vi "Fluke 5080 Resistance Calibrator.vi"() -> ()   [LabVIEW 2012]
doc: "This example shows how to configure the calibrator to resistance output mode."
uses:
  <instrlib>/Fluke 5080/Fluke 5080.lvlib
panel:
  in  "Resistance (1900.0 Ohm)":dbl=1900.0
  in  "Impedance Compensation (0: None)":i32(ring) items=["None", "2-wire", "4-wire"]
  in  "Serial Configuration":T1={"Baud Rate"=9600, "Parity"=0, "Data Bits"=8, "Stop Bits"=10, "Flow Control"=0} {"Flow Control" items=["None", "XON/XOFF", "RTS/CTS", "XON/XOFF & RTS/CTS", "DTR/DSR", "XON/XOFF & DTR/DSR"]; "Stop Bits" items=["1.0"=10, "1.5"=15, "2.0"=20]; "Data Bits" items=["7"=7, "8"=8]; "Parity" items=["None", "Odd", "Even", "Mark", "Space"]; "Baud Rate" items=["300"=300, "600"=600, "1200"=1200, "2400"=2400, "4800"=4800, "9600"=9600, "19200"=19200]}
  in  "VISA resource name":refnum<visa-resource-name>
  in  "Output Type (0: DC Volts)":i32(ring)=8 items=["DC Volts", "AC Volts", "DC Current", "AC Current", "DC Power", "AC Power", "Dual DC Volts", "Dual AC Volts", "Resistance"]
  # "(c) 2010 National Instruments.  ALL RIGHTS RESERVED."
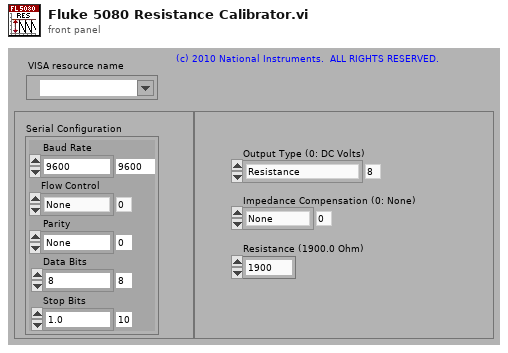
[diagram p1: front panel]
types:
  T1 = cluster{"Baud Rate":u32, "Parity":u16, "Data Bits":u16, "Stop Bits":u16, "Flow Control":u16}
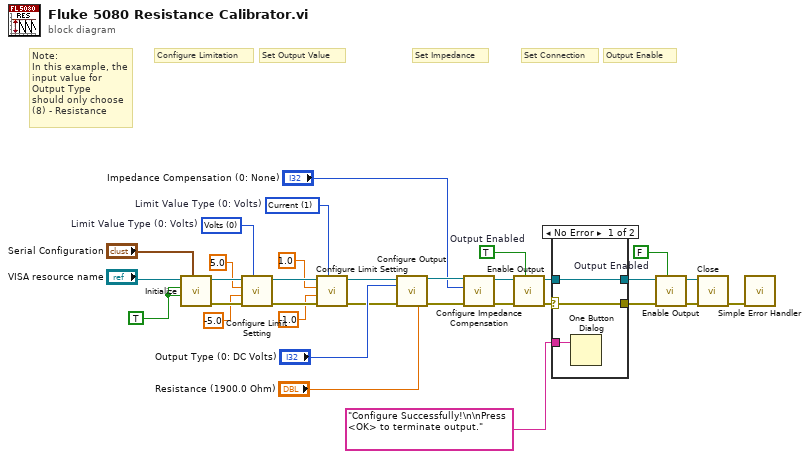
[diagram p0: block diagram]
diagram:
  w5 = 1 items=["Volts", "Current"]  # Limit Value Type (0: Volts)
  w6 = 0 items=["Volts", "Current"]  # Limit Value Type (0: Volts)
  w11 = TRUE  # Output Enabled
  w19 = FALSE  # Output Enabled
  w32 = TRUE ("Reset (True)")
  # "Set Connection"
  # "Note:\nIn this example, the \ninput value for \nOutput Type\nshould only choose \n(8) - Resistance"
  # "Output Enable"
  # "Set Impedance"
  # "Set Output Value"
  # "Configure Limitation"
  n1 = call <instrlib>:"Initialize.vi"("Serial Configuration"="Serial Configuration", "Reset (True)"=w32, "ID Query (True)"=w32, "VISA resource name"="VISA resource name") -> ("error out"=w31:errorcluster, "VISA resource name out"=w30:refnum<visa-resource-name>)  [unwired: 1 in, 5 out]
  n2 = call <instrlib>:"Configure Limit Setting.vi"("Limit Value Type (0: Volts)"=w6, "error in (no error)"=w31, "- Limit Value (-5)"=-5.0, "+ Limit Value (5)"=5.0, "VISA resource name"=w30) -> ("error out"=w9:errorcluster, "VISA resource name out"=w10:refnum<visa-resource-name>)  [unwired: 5 out]
  n3 = call <instrlib>:"Configure Limit Setting.vi"("Limit Value Type (0: Volts)"=w5, "error in (no error)"=w9, "- Limit Value (-5)"=-1.0, "+ Limit Value (5)"=1.0, "VISA resource name"=w10) -> ("error out"=w7:errorcluster, "VISA resource name out"=w8:refnum<visa-resource-name>)  [unwired: 5 out]
  n4 = call <instrlib>:"Configure Output.vi"("VISA resource name"=w8, "Resistance (1900.0 Ohm)"="Resistance (1900.0 Ohm)", "Output Type (0: DC Volts)"="Output Type (0: DC Volts)", "error in (no error)"=w7) -> ("VISA resource name out"=w25:refnum<visa-resource-name>, "error out"=w24:errorcluster)  [unwired: 6 in, 4 out]
  n5 = call <instrlib>:"Configure Impedance Compensation.vi"("error in (no error)"=w24, "Impedance Compensation (0: None)"="Impedance Compensation (0: None)", "VISA resource name"=w25) -> ("error out"=w20:errorcluster, "VISA resource name out"=w21:refnum<visa-resource-name>)  [unwired: 7 out]
  n6 = call <instrlib>:"Enable Output.vi"("Output Enabled (T: Enable)"=w11, "error in (no error)"=w20, "VISA resource name"=w21) -> ("error out"=w12:errorcluster, "VISA resource name out"=w13:refnum<visa-resource-name>)  [unwired: 7 out]
  n7 = case shown="No Error" w12 {
    selector: w12 -> [w34 w36]
    tunnel: "Configure Successfully!\n\nPress <OK> to terminate output." ("message") -> [w35 _]
    tunnel: [w34 w36] -> w16
    tunnel: [w33 w37] -> w17
    tunnel: w13 -> [w33 w37]
    frame No Error {
      n8 = One Button Dialog(message=w35) -> ()  [unwired: 2 out]
    }
    frame Error {
    }
  }
  n9 = call <instrlib>:"Enable Output.vi"("Output Enabled (T: Enable)"=w19, "error in (no error)"=w16, "VISA resource name"=w17) -> ("error out"=w14:errorcluster, "VISA resource name out"=w15:refnum<visa-resource-name>)  [unwired: 7 out]
  n10 = call <instrlib>:"Close.vi"("error in (no error)"=w14, "VISA resource name"=w15) -> ("error out"=w29:errorcluster)  [unwired: 9 out]
  n11 = call <vilib>:"Simple Error Handler.vi"("error in (no error)"=w29) -> ()  [unwired: 1 in, 8 out]
